vi "Create StringList.vi"(7 "List Implementation (Array)":refnum<class "ListImp.lvclass">, 8 "error in (no error)":errorcluster) -> (0 "error out":errorcluster, 3 "StringList out":refnum<class "StringList.lvclass">)   [LabVIEW 2017, in "LapDog.Collections.v0.Lists.Interfaces.lvlib" / "StringList.lvclass"]
uses:
  StringList.lvclass
  Lists/ListImp/ListImp.lvclass
  StringList.lvclass/StringList.ctl
  Lists/List/List.lvclass
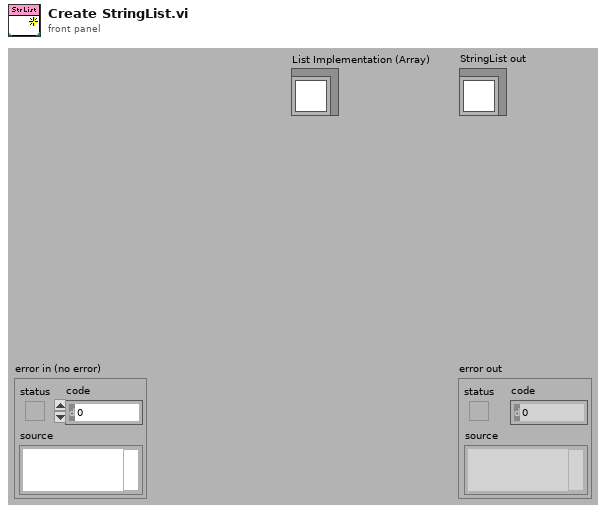
[diagram p1: front panel]
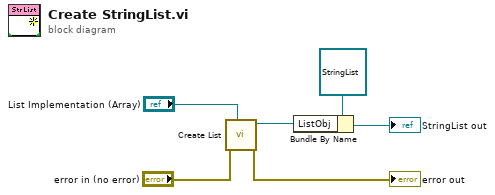
[diagram p0: block diagram]
diagram:
  n1 = call "Create List.vi"("List Implementation (Array)"="List Implementation (Array)", "error in (no error)"="error in (no error)") -> ("error out"=→"error out":errorcluster, "List out"=w4:refnum<class "List.lvclass">)  [unwired: 8 in]
  n2 = Bundle By Name(cluster=refnum<class "StringList.lvclass"> refnum ("StringList in"), "ListObj"=w4) -> (→"StringList out":refnum<class "StringList.lvclass">)
